vi "PRIME Detector Read TCP Response.vi"(8 "error in (no error)":errorcluster, 10 "timeout ms (6000)":i32=6000, 11 "connection ID":refnum<k5>) -> (0 "error out":errorcluster, 1 "prefix":string, 2 "response message":string, 3 "connection ID out":refnum<k5>)   [LabVIEW 2021, in "PRIME Detector.lvclass"]
uses:
  PRIME Detector.lvclass
panel:
  out "Size":u32
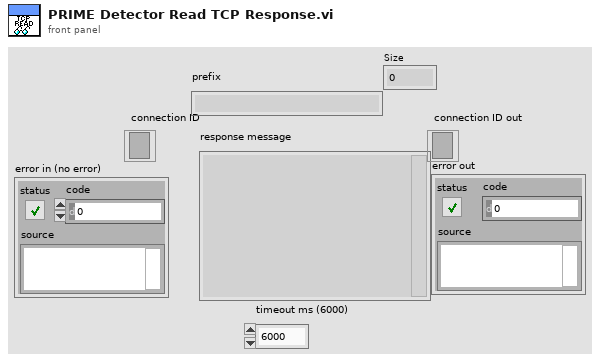
[diagram p1: front panel]
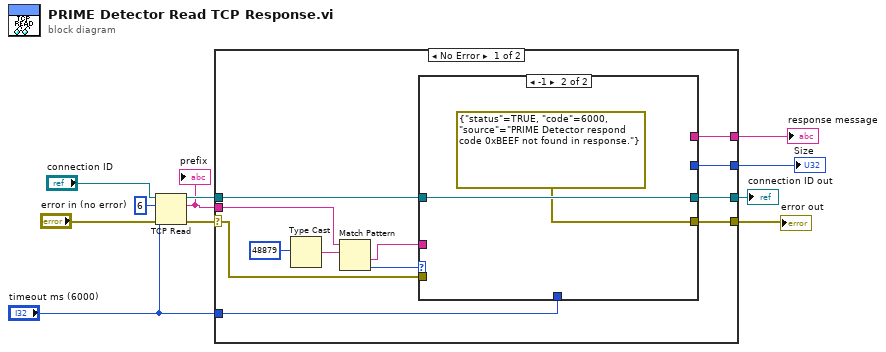
[diagram p0: block diagram]
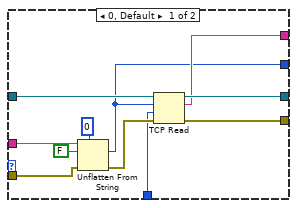
[diagram p2: hidden frame]
diagram:
  n1 = TCP Read(connection ID="connection ID", bytes to read=6, error in (no error)="error in (no error)", 9:"timeout ms (6000)") -> (connection ID out=w9:refnum<k5>, data out=w8:string, error out=w10:errorcluster)  [unwired: 1 in]
  "prefix" <- w8
  n2 = case shown="No Error" w10 {
    selector: w10 -> [w19 w38]
    tunnel: w9 -> [w18 w37]
    tunnel: w8 -> [w21 _]
    tunnel: "timeout ms (6000)" -> [w17 _]
    tunnel: [w16 w38] -> w6
    tunnel: [w15 w37] -> w4
    tunnel: [w14 _] -> w3
    tunnel: [w12 _] -> w1
    frame No Error {
      n3 = Type Cast(x=u16 48879) -> (*(type *) &x=w23:string)  [unwired: 1 in]
      n4 = Match Pattern(string=w21, regular expression=w23) -> (after substring=w20:string, offset past match=w13:i32)  [unwired: 1 in, 2 out]
      n5 = case shown="-1" w13 {
        tunnel: w20 -> [w34 _]
        tunnel: w19 -> [w31 _]
        tunnel: w18 -> [w30 w36]
        tunnel: w17 -> [w28 _]
        tunnel: [w27 errorcluster {"status"=TRUE, "code"=6000, "source"="PRIME Detector respond code 0xBEEF not found in response."} ("error out")] -> w16
        tunnel: [w26 w36] -> w15
        tunnel: [w25 _] -> w14
        tunnel: [w24 _] -> w12
        frame 0, Default {
          n6 = Unflatten From String(type=u32 0, binary string=w34, data includes array or string size? (T)=FALSE, error in (no error)=w31) -> (value=w24:u32, error out=w29:errorcluster)  [unwired: 1 in, 1 out]
          n7 = TCP Read(connection ID=w30, bytes to read=w24, error in (no error)=w29, 9:w28) -> (connection ID out=w26:refnum<k5>, data out=w25:string, error out=w27:errorcluster)  [unwired: 1 in]
        }
        frame -1 {
        }
      }
    }
    frame Error {
    }
  }
  "connection ID out" <- w4
  "error out" <- w6
  "response message" <- w3
  "Size" <- w1
